vi "MultiTableGenerateData.vi"(8 "error in (no error)":errorcluster, 11 "Cluster Variant":variant) -> (0 "error out":errorcluster, 3 "Data":string[][](array[string]))   [LabVIEW 2014, in "TableLogger_Actor.lvlib" / "TableLogger_Actor.lvclass"]
uses:
  TableLogger_Actor.lvclass
panel:
  # "Connector Pane"
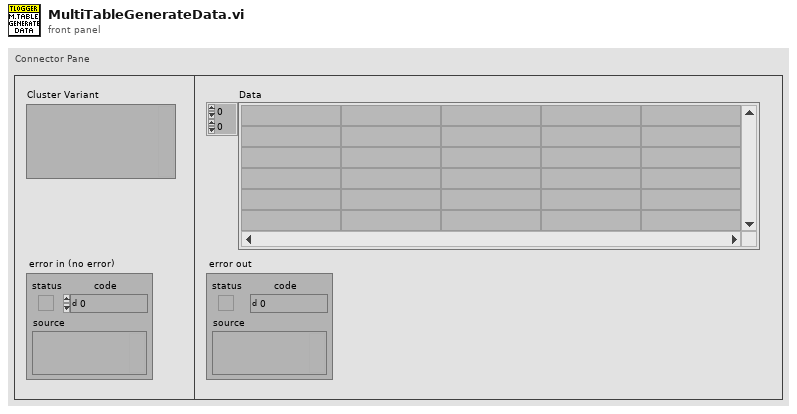
[diagram p1: front panel]
types:
  T1 = typedef "Type Descriptor Enumeration__ogtk.ctl" = enum8{"<Null>", "I8", "I16", "I32", "I64", "U8", "U16", "U32", "U64", "SGL", "DBL", "EXT", "CSG", "CDB", "CXT", "0x0F", "0x10", "0x11", "0x12", "0x13", "0x14", "Enum U8", "Enum U16", "Enum U32", "Enum U64", "SGL PQ", "DBL PQ", "EXT PQ", "CSG PQ", "CDB PQ", "CXT PQ", "0x1F", "0x20", "Boolean", "0x22", "0x23", "0x24", "0x25", "0x26", "0x27", "0x28", "0x29", "0x2A", "0x2B", "0x2C", "0x2D", "0x2E", "0x2F", "String", "0x31", "Path", "Pict", "0x34", "0x35", "0x36", "DAQ", "0x38", "0x39", "0x3A", "0x3B", "0x3C", "0x3D", "0x3E", "0x3F", "Array", "0x41", "0x42", "0x43", "0x44", "0x45", "0x46", "0x47", "0x48", "0x49", "0x4A", "0x4B", "0x4C", "0x4D", "0x4E", "0x4F", "Cluster", "0x51", "0x52", "Variant", "Waveform", "0x55", "0x56", "0x57", "0x58", "0x59", "0x5A", "0x5B", "0x5C", "0x5D", "0x5E", "0x5F", "0x60", "0x61", "0x62", "0x63", "0x64", "0x65", "0x66", "0x67", "0x68", "0x69", "0x6A", "0x6B", "0x6C", "0x6D", "0x6E", "0x6F", "Refnum"}
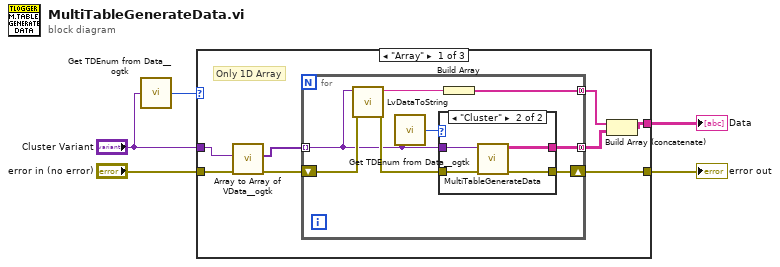
[diagram p0: block diagram]
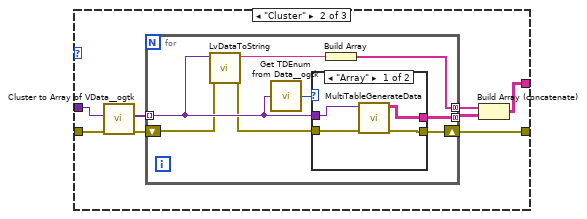
[diagram p3: hidden frame]
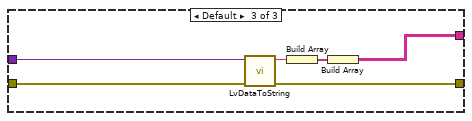
[diagram p5: hidden frame]
diagram:
  n1 = call <userlib>:"Get TDEnum from Data__ogtk.vi"("Data"="Cluster Variant") -> ("Type Descriptor Enumeration"=w1:T1)  [unwired: 4 in]
  n2 = case shown="\"Array\"" w1 {
    tunnel: "Cluster Variant" -> [w13 w33 w48]
    tunnel: [w7 w28 w51] -> w5
    tunnel: "error in (no error)" -> [w12 w31 w50]
    tunnel: [w9 w29 w49] -> w4
    frame "Array" {
      # "Only 1D Array"
      n3 = call <userlib>:"Array to Array of VData__ogtk.vi"("error in (no error)"=w12, "MultiD Array"=w13) -> ("error out"=w10:errorcluster, "1D Array of Variants"=w11:variant[])  [unwired: 8 in]
      n4 = for {
        tunnel: w11 -> [w16] mode=indexing
        tunnel: [w19] -> w8 mode=concatenating
        shift-right: [w17] -> w9
        shift-left: w10 -> [w21]
        tunnel: [w14] -> w6 mode=concatenating
        n5 = call "LvDataToString.vi"("error in (no error)"=w21, "Variant"=w16) -> ("error out"=w18:errorcluster, "String Value"=w20:string)  [unwired: 8 in]
        n6 = call <userlib>:"Get TDEnum from Data__ogtk.vi"("Data"=w16) -> ("Type Descriptor Enumeration"=w15:T1)  [unwired: 4 in]
        n7 = case shown="\"Cluster\"" w15 {
          tunnel: w16 -> [_ w26]
          tunnel: w18 -> [w22 w25]
          tunnel: [w22 w24] -> w17
          tunnel: [_ w23] -> w14
          frame "<Null>", Default {
          }
          frame "Cluster" {
            n8 = call "MultiTableGenerateData.vi"("error in (no error)"=w25, "Cluster Variant"=w26) -> ("error out"=w24:errorcluster, "Data"=w23:string[][])  [unwired: 8 in]
          }
        }
        n9 = Build Array(w20) -> (w19:string[])
      }
      n10 = Build Array (concatenate)(w8, w6) -> (w7:string[][])
    }
    frame "Cluster" {
      n11 = call <userlib>:"Cluster to Array of VData__ogtk.vi"("error in (no error)"=w31, "Cluster"=w33) -> ("error out"=w30:errorcluster, "Array of VData"=w32:variant[])  [unwired: 8 in]
      n12 = for {
        tunnel: w32 -> [w40] mode=indexing
        tunnel: [w36] -> w34 mode=concatenating
        shift-right: [w42] -> w29
        shift-left: w30 -> [w39]
        tunnel: [w35] -> w27 mode=concatenating
        n13 = call "LvDataToString.vi"("error in (no error)"=w39, "Variant"=w40) -> ("error out"=w38:errorcluster, "String Value"=w37:string)  [unwired: 8 in]
        n14 = call <userlib>:"Get TDEnum from Data__ogtk.vi"("Data"=w40) -> ("Type Descriptor Enumeration"=w41:T1)  [unwired: 4 in]
        n15 = case shown="\"Array\"" w41 {
          tunnel: w40 -> [w46 _]
          tunnel: w38 -> [w45 w47]
          tunnel: [w44 w47] -> w42
          tunnel: [w43 _] -> w35
          frame "Array" {
            n16 = call "MultiTableGenerateData.vi"("error in (no error)"=w45, "Cluster Variant"=w46) -> ("error out"=w44:errorcluster, "Data"=w43:string[][])  [unwired: 8 in]
          }
          frame Default {
          }
        }
        n17 = Build Array(w37) -> (w36:string[])
      }
      n18 = Build Array (concatenate)(w34, w27) -> (w28:string[][])
    }
    frame Default {
      n19 = call "LvDataToString.vi"("error in (no error)"=w50, "Variant"=w48) -> ("error out"=w49:errorcluster, "String Value"=w53:string)  [unwired: 8 in]
      n20 = Build Array(w53) -> (w52:string[])
      n21 = Build Array(w52) -> (w51:string[][])
    }
  }
  "Data" <- w5
  "error out" <- w4
